vi "PH_Powermeter_BaseClass.PC Set Wavelength.vi"(0 "VI in":refnum<vi>, 2 "Wanted Wavelength [nm]":u32=1, 5 "error in (no error)":errorcluster) -> (14 "VI out":refnum<vi>, 19 "error out":errorcluster)   [LabVIEW 2014, in "PH_Powermeter_BaseClass.lvlib"]
doc: "If the incoming value is not zero and deiffers from stored value, the scaling factor is set to own attributtes. Aferwards, the energy is recalculated and set as well to own attributes as to GUI and DIM service."
uses:
  PH_Powermeter_BaseClass.lvlib
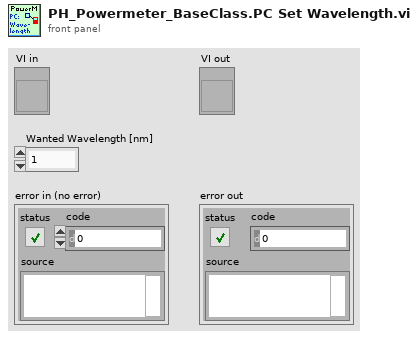
[diagram p1: front panel]
types:
  T1 = typedef "PH_Powermeter_BaseClass.lvlib/PH_Powermeter_BaseClass.i attribute.ctl" = cluster{"GUI References":T2, "Connection":T3, "Head Attributes":T5, "VISA resource":refnum<visa-resource-name>, "Energy":T6, "Service ID Energy":i32, "Wanted Settings":T7, "Current Settings":T7}
  T2 = typedef "PH_Powermeter_BaseClass.lvlib/PH_Powermeter_BaseClass.GUI Refs.ctl" = cluster{"Head Attributes":refnum<vi>, "Energy":refnum<vi>, "Connection":refnum<vi>, "VISA Resource":refnum<vi>, "Scaling Factor":refnum<vi>, "Range":refnum<vi>, "Wavelength":refnum<vi>, "Trigger Level":refnum<vi>, "Wanted Settings":refnum<vi>, "Current Settings":refnum<vi>}
  T3 = typedef "PH_Powermeter_BaseClass.lvlib/PH_Powermeter_BaseClass.Connection.ctl" = cluster{"failed checks":i8, "Timeout":bool, "Data read":string, "Failure":bool, "Error":bool, "State":T4}
  T4 = typedef "PH_Powermeter_BaseClass.lvlib/PH_Powermeter_BaseClass.State.ctl" = enum32{"off", "operating", "opened", "checked", "connected", "Sets to change", "running"}
  T5 = typedef "PH_Powermeter_BaseClass.lvlib/PH_Powermeter_BaseClass.Head Attributes.ctl" = cluster{"Instrument Type":string, "Head Version":string, "Head Name":string, "Serial Number":string, "Firmware":string, "Sensor Type":string, "MinimumRange":u32, "Maximum Range":u32, "Min Wavelength":i32, "Max Wavelength":i32}
  T6 = typedef "PH_Powermeter_BaseClass.lvlib/PH_Powermeter_BaseClass.Energy.ctl" = cluster{"current Value":dbl, "unscaled":dbl, "Scaling Factor":dbl}
  T7 = typedef "PH_Powermeter_BaseClass.lvlib/PH_gentec_BaseClass.Head Settings.ctl" = cluster{"Trigger Level":dbl, "Wavelength":u32, "Range":u32}
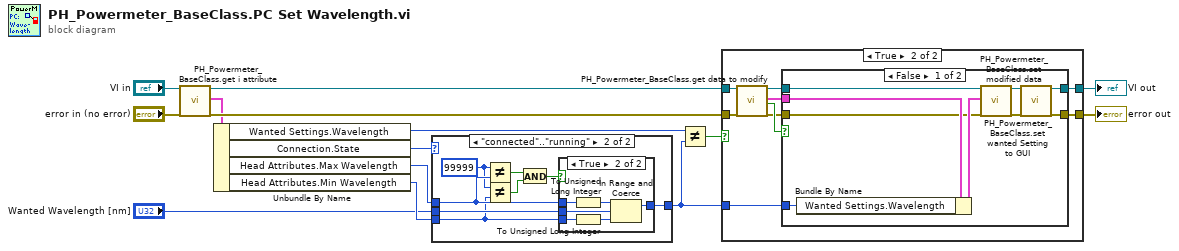
[diagram p0: block diagram]
diagram:
  n1 = call "PH_Powermeter_BaseClass.get i attribute.vi"("i ref in"="VI in", "error in (no error)"="error in (no error)") -> ("i ref out"=w9:refnum<vi>, "i attribute"=w8:T1, "error out"=w10:errorcluster)  [unwired: 15 in]
  n2 = Unbundle By Name(w8) -> ("Wanted Settings.Wavelength"=w7:u32, "Connection.State"=w1:T4, "Head Attributes.Max Wavelength"=w5:i32, "Head Attributes.Min Wavelength"=w4:i32)
  n3 = case shown="\"connected\"..\"running\"" w1 {
    tunnel: w5 -> [_ w21]
    tunnel: w4 -> [_ w20]
    tunnel: "Wanted Wavelength [nm]" -> [w15 w23]
    tunnel: [w15 w22] -> w2
    frame "off", Default {
    }
    frame "connected".."running" {
      w19 = 99999 ("x")
      n4 = Not Equal?(x=w19, y=w21) -> (x != y?=w18:bool)
      n5 = Not Equal?(x=w19, y=w20) -> (x != y?=w17:bool)
      n6 = And(x=w18, y=w17) -> (x .and. y?=w16:bool)
      n7 = case shown="True" w16 {
        tunnel: w23 -> [w24 w30]
        tunnel: [w24 w29] -> w22
        tunnel: w21 -> [_ w26]
        tunnel: w20 -> [_ w25]
        frame False {
        }
        frame True {
          n8 = To Unsigned Long Integer(number=w26) -> (unsigned 32bit integer=w28:u32)
          n9 = To Unsigned Long Integer(number=w25) -> (unsigned 32bit integer=w27:u32)
          n10 = In Range and Coerce(upper limit=w28, x=w30, lower limit=w27) -> (coerced(x)=w29:u32)  [unwired: 1 out]
        }
      }
    }
  }
  n11 = Not Equal?(x=w7, y=w2) -> (x != y?=w6:bool)
  n12 = case shown="True" w6 {
    tunnel: [w31 w39] -> w14
    tunnel: [w32 w37] -> w12
    tunnel: w10 -> [w31 w35]
    tunnel: w9 -> [w32 w34]
    tunnel: w2 -> [_ w33]
    frame False {
    }
    frame True {
      n13 = call "PH_Powermeter_BaseClass.get data to modify.vi"("i ref in"=w34, "error in (no error)"=w35) -> ("i ref out"=w36:refnum<vi>, "i attribute"=w41:T1, "timed out"=w40:bool, "error out"=w38:errorcluster)  [unwired: 14 in]
      n14 = case shown="False" w40 {
        tunnel: w36 -> [w50 w52]
        tunnel: [w42 w52] -> w37
        tunnel: w38 -> [w46 w51]
        tunnel: [w44 w51] -> w39
        tunnel: w41 -> [w48 _]
        tunnel: w33 -> [w47 _]
        frame False {
          n15 = Bundle By Name(cluster=w48, "Wanted Settings.Wavelength"=w47) -> (w49:T1)
          n16 = call "PH_Powermeter_BaseClass.set modified data.vi"("i ref in"=w50, "i attribute"=w49, "error in (no error)"=w46) -> ("i ref out"=w43:refnum<vi>, "error out"=w45:errorcluster)  [unwired: 15 in]
          n17 = call "PH_Powermeter_BaseClass.set wanted Setting to GUI.vi"("VI in"=w43, "error in (no error)"=w45) -> ("VI out"=w42:refnum<vi>, "error out"=w44:errorcluster)  [unwired: 16 in]
        }
        frame True {
        }
      }
    }
  }
  "error out" <- w14
  "VI out" <- w12
